vi "Viewer speed UI interface.vi"(5 "Caller":enum16{"Viewer", "Exporter"}(ring), 6 "Funct data structure":bool, 7 "Function":enum16{"Initialise", "Update"}(ring), 8 "error in (no error)":errorcluster, 9 "Gobal frame number in Timelapse data/master video (1 based)":i32=1, 10 "Number of Frames":u32, 11 "Speed Data folder path+dummy filename":path) -> (0 "error out":errorcluster, 1 "Speed Data":string[][](array[string]), 3 "Actual number of speed values":i32, 4 "Speed waveform graph data":dbl[](array[numeric]))   [LabVIEW 2013]
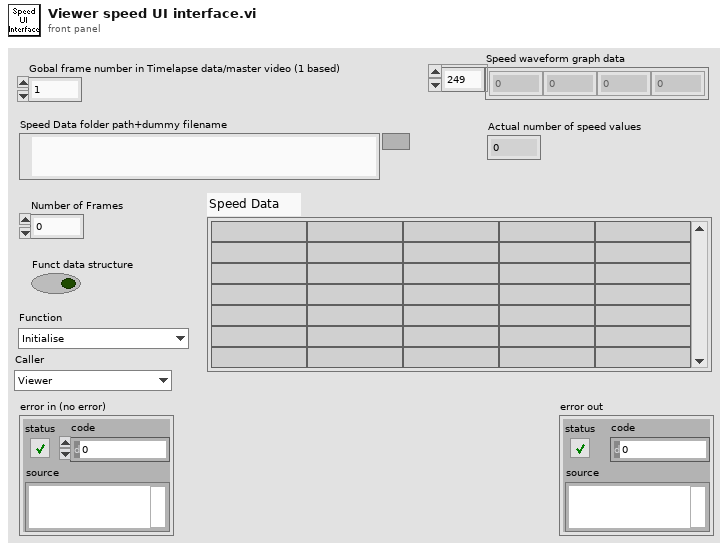
[diagram p1: front panel]
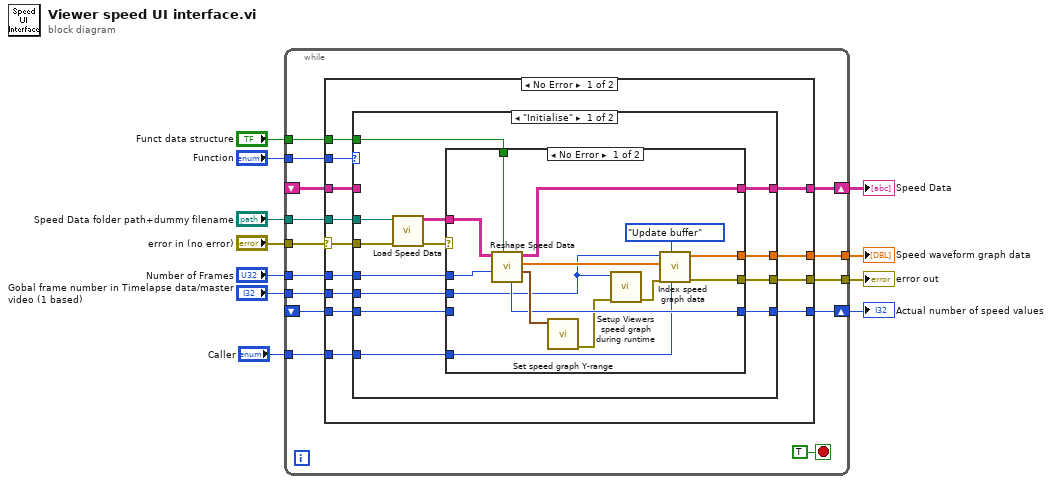
[diagram p0: block diagram]
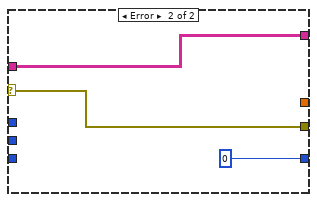
[diagram p2: hidden frame]
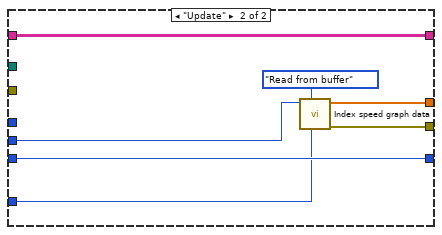
[diagram p3: hidden frame]
diagram:
  n1 = while {
    tunnel: "Number of Frames" -> [w25]
    tunnel: "Speed Data folder path+dummy filename" -> [w24]
    tunnel: [w22] -> w8
    tunnel: "error in (no error)" -> [w16]
    tunnel: [w20] -> w4
    tunnel: "Gobal frame number in Timelapse data/master video (1 based)" -> [w19]
    tunnel: "Function" -> [w18]
    shift-right: [w21] -> w7
    shift-left: _ -> [w15]
    shift-right: [w23] -> w9
    shift-left: _ -> [w14]
    tunnel: "Funct data structure" -> [w13]
    tunnel: "Caller" -> [w12]
    stop <- TRUE stop-if-true
    n2 = case shown="No Error" w16 {
      selector: w16 -> [w30 w78]
      tunnel: w25 -> [w38 _]
      tunnel: w24 -> [w37 _]
      tunnel: [w36 w76] -> w23
      tunnel: [w35 w78] -> w22
      tunnel: [w34 w77] -> w21
      tunnel: [w33 _] -> w20
      tunnel: w19 -> [w32 _]
      tunnel: w18 -> [w31 _]
      tunnel: w15 -> [w28 w77]
      tunnel: w14 -> [w29 w76]
      tunnel: w13 -> [w27 _]
      tunnel: w12 -> [w26 _]
      frame No Error {
        n3 = case shown="\"Initialise\"" w31 {
          tunnel: w38 -> [w51 _]
          tunnel: w37 -> [w50 _]
          tunnel: [w49 w70] -> w36
          tunnel: [w48 w75] -> w35
          tunnel: [w47 w71] -> w34
          tunnel: w30 -> [w46 _]
          tunnel: [w45 w74] -> w33
          tunnel: w32 -> [w44 w73]
          tunnel: w29 -> [w41 w70]
          tunnel: w28 -> [_ w71]
          tunnel: w27 -> [w40 _]
          tunnel: w26 -> [w39 w69]
          frame "Initialise" {
            n4 = call "Load Speed Data.vi"("error in (no error)"=w46, "AVI File Path"=w50) -> ("error out"=w43:errorcluster, "Speed Data"=w42:string[][])  [unwired: 8 in]
            n5 = case shown="No Error" w43 {
              selector: w43 -> [_ w68]
              tunnel: w51 -> [w57 _]
              tunnel: [w62 0 ("Output number of speed points \n(after interpolation)")] -> w49
              tunnel: w42 -> [w64 w67]
              tunnel: [w60 w68] -> w48
              tunnel: [w63 w67] -> w47
              tunnel: [w61 _] -> w45
              tunnel: w44 -> [w52 _]
              tunnel: w41 -> [_ _]
              tunnel: w40 -> [w56 _]
              tunnel: w39 -> [w55 _]
              frame No Error {
                n6 = call "Reshape Speed Data.vi"("Funct data structure"=w56, "Number of time series microscope data frames"=w57, "all rows"=w64) -> ("Speed max/min"=w65:cluster{"max value":dbl, "min value":dbl}, "Averaged CM/SEC speeds array (one speed value per image frame)"=w58:dbl[], "Speed Data"=w63:string[][], "Output number of speed points \n(after interpolation)"=w62:i32)  [unwired: 3 in, 2 out]
                n7 = call "Set speed graph Y-range.vi"("Speed max/min"=w65) -> ("error out"=w53:errorcluster)  [unwired: 10 in]
                n8 = call "Setup Viewers speed graph during runtime.vi"("error in (no error)"=w53, "Frame number"=w52) -> ("error out"=w54:errorcluster)  [unwired: 9 in]
                n9 = call "Index speed graph data.vi"("Caller"=w55, "Buffer operation (read from internal buffer)"=enum16{"Update buffer", "Read from buffer"}."Update buffer" ("Buffer operation"), "error in (no error)"=w54, "Averaged speeds (one per frame)"=w58, "Gobal frame number in Timelapse data/master video (1 based)"=w52) -> ("error out"=w60:errorcluster, "Speed data waveform graph"=w61:dbl[])  [unwired: 4 in, 1 out]
              }
              frame Error {
              }
            }
          }
          frame "Update" {
            n10 = call "Index speed graph data.vi"("Caller"=w69, "Buffer operation (read from internal buffer)"=enum16{"Update buffer", "Read from buffer"}."Read from buffer" ("Buffer operation"), "Gobal frame number in Timelapse data/master video (1 based)"=w73) -> ("error out"=w75:errorcluster, "Speed data waveform graph"=w74:dbl[])  [unwired: 6 in, 1 out]
          }
        }
      }
      frame Error {
      }
    }
  }
  "Speed Data" <- w7
  "Actual number of speed values" <- w9
  "error out" <- w8
  "Speed waveform graph data" <- w4
